vi "trim_string_of_wspaces_and_quotes.vi"(4 "String in":string, 5 "Remove quotes (Remove All)":u16(ring) items=["Remove All Quotes", "Remove Single Quotes", "Remove Double Quotes", "Remove None"]) -> (1 "String out":string)   [LabVIEW 2014, in "rszvl_rsidr_core.lvlib"]
uses:
  rszvl_rsidr_core.lvlib
  Match Regular Expression.xnode
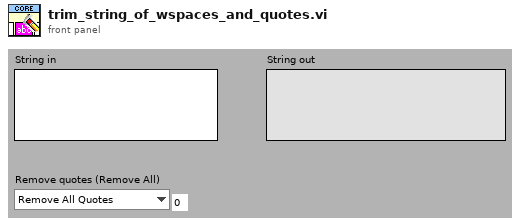
[diagram p1: front panel]
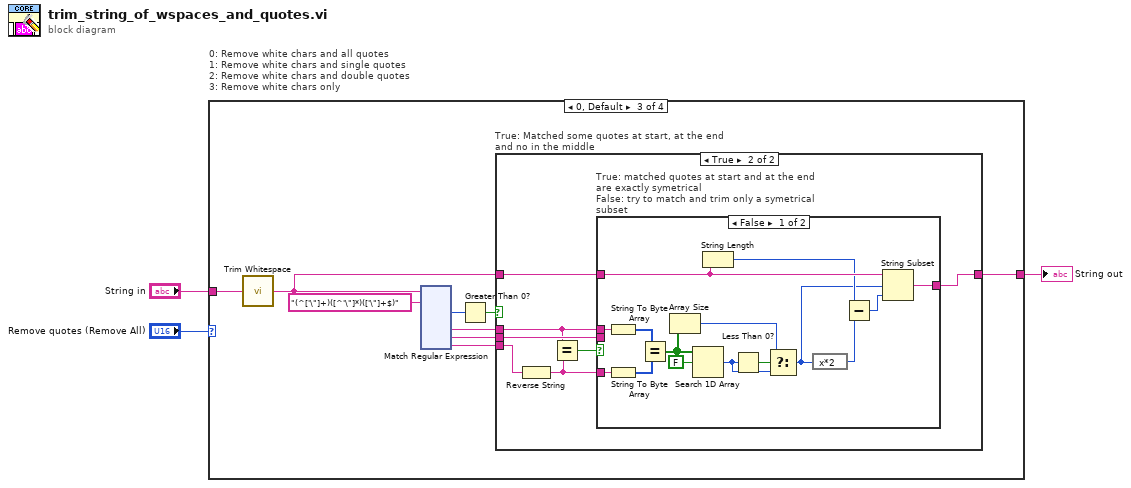
[diagram p0: block diagram]
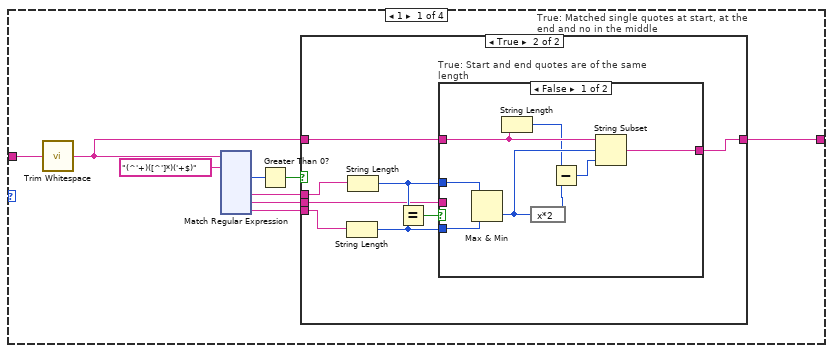
[diagram p2: hidden frame]
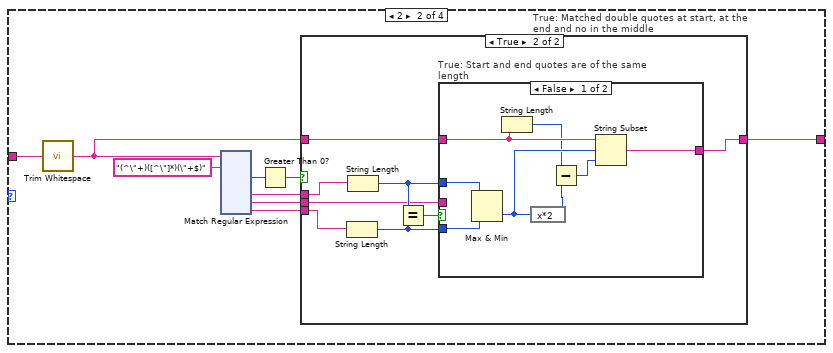
[diagram p5: hidden frame]
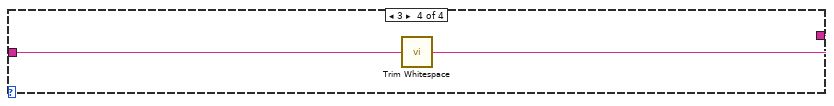
[diagram p10: hidden frame]
diagram:
  n1 = case "0: Remove white chars and all quotes\n1: Remove white chars and single quotes\n2: Remove white chars and double quotes\n3: Remove white chars only" shown="0, Default" "Remove quotes (Remove All)" {
    tunnel: "String in" -> [w12 w154 w296 w437]
    tunnel: [w5 w148 w288 w436] -> w1
    frame 1 {
      n2 = call "Trim Whitespace.vi"("string"=w12) -> ("trimmed string"=w4:string)  [unwired: 1 in]
      n3 = xnode ("Match Regular Expression")("input string"=w4, "regular expression"="(^'+)([^']*)('+$)") -> ("offset past match"=w10:i32, "submatch 1"=w8:string, "submatch 2"=w7:string, "submatch 3"=w6:string)  [unwired: 4 in, 4 out]
      n4 = Greater Than 0?(x=w10) -> (x > 0?=w9:bool)
      n5 = case "True: Matched single quotes at start, at the end and no in the middle" shown="True" w9 {
        tunnel: w8 -> [_ w20]
        tunnel: w7 -> [_ w16]
        tunnel: w6 -> [_ w21]
        tunnel: [w13 w15] -> w5
        tunnel: w4 -> [w13 w14]
        frame False {
        }
        frame True {
          n6 = String Length(string=w21) -> (length=w17:i32)
          n7 = String Length(string=w20) -> (length=w18:i32)
          n8 = Equal?(x=w18, y=w17) -> (x = y?=w19:bool)
          n9 = case "True: Start and end quotes are of the same length" shown="False" w19 {
            tunnel: w18 -> [w29 _]
            tunnel: w17 -> [w28 _]
            tunnel: w16 -> [_ w30]
            tunnel: [w22 w30] -> w15
            tunnel: w14 -> [w27 _]
            frame False {
              n10 = Max & Min(x=w29, y=w28) -> (min(x,y)=w26:i32)  [unwired: 1 out]
              n11 = String Length(string=w27) -> (length=w25:i32)
              n12 = expression code="x*2"(w26) -> (w24:i32)
              n13 = Subtract(x=w25, y=w24) -> (x-y=w23:i32)
              n14 = String Subset(string=w27, offset (0)=w26, length (rest)=w23) -> (substring=w22:string)
            }
            frame True {
            }
          }
        }
      }
    }
    frame 2 {
      n15 = call "Trim Whitespace.vi"("string"=w154) -> ("trimmed string"=w147:string)  [unwired: 1 in]
      n16 = xnode ("Match Regular Expression")("input string"=w147, "regular expression"="(^\"+)([^\"]*)(\"+$)") -> ("offset past match"=w153:i32, "submatch 1"=w151:string, "submatch 2"=w150:string, "submatch 3"=w149:string)  [unwired: 4 in, 4 out]
      n17 = Greater Than 0?(x=w153) -> (x > 0?=w152:bool)
      n18 = case "True: Matched double quotes at start, at the end and no in the middle" shown="True" w152 {
        tunnel: w151 -> [_ w162]
        tunnel: w150 -> [_ w158]
        tunnel: w149 -> [_ w163]
        tunnel: [w155 w157] -> w148
        tunnel: w147 -> [w155 w156]
        frame False {
        }
        frame True {
          n19 = String Length(string=w163) -> (length=w159:i32)
          n20 = String Length(string=w162) -> (length=w160:i32)
          n21 = Equal?(x=w160, y=w159) -> (x = y?=w161:bool)
          n22 = case "True: Start and end quotes are of the same length" shown="False" w161 {
            tunnel: w160 -> [w171 _]
            tunnel: w159 -> [w170 _]
            tunnel: w158 -> [_ w172]
            tunnel: [w164 w172] -> w157
            tunnel: w156 -> [w169 _]
            frame False {
              n23 = Max & Min(x=w171, y=w170) -> (min(x,y)=w168:i32)  [unwired: 1 out]
              n24 = String Length(string=w169) -> (length=w167:i32)
              n25 = expression code="x*2"(w168) -> (w166:i32)
              n26 = Subtract(x=w167, y=w166) -> (x-y=w165:i32)
              n27 = String Subset(string=w169, offset (0)=w168, length (rest)=w165) -> (substring=w164:string)
            }
            frame True {
            }
          }
        }
      }
    }
    frame 0, Default {
      n28 = call "Trim Whitespace.vi"("string"=w296) -> ("trimmed string"=w289:string)  [unwired: 1 in]
      n29 = xnode ("Match Regular Expression")("input string"=w289, "regular expression"="(^['\"]+)([^'\"]*)(['\"]+$)") -> ("offset past match"=w294:i32, "submatch 1"=w292:string, "submatch 2"=w291:string, "submatch 3"=w290:string)  [unwired: 4 in, 4 out]
      n30 = Greater Than 0?(x=w294) -> (x > 0?=w293:bool)
      n31 = case "True: Matched some quotes at start, at the end and no in the middle" shown="True" w293 {
        tunnel: w292 -> [_ w298]
        tunnel: w291 -> [_ w303]
        tunnel: w290 -> [_ w300]
        tunnel: [w297 w302] -> w288
        tunnel: w289 -> [w297 w301]
        frame False {
        }
        frame True {
          n32 = Reverse String(1:w300) -> (0:w299:string)
          n33 = Equal?(x=w298, y=w299) -> (x = y?=w304:bool)
          n34 = case "True: matched quotes at start and at the end are exactly symetrical\nFalse: try to match and trim only a symetrical subset" shown="False" w304 {
            tunnel: w303 -> [_ w320]
            tunnel: [w316 w320] -> w302
            tunnel: w301 -> [w319 _]
            tunnel: w299 -> [w314 _]
            tunnel: w298 -> [w315 _]
            frame False {
              n35 = String To Byte Array(string=w315) -> (unsigned byte array=w313:u8[])
              n36 = String To Byte Array(string=w314) -> (unsigned byte array=w312:u8[])
              n37 = Equal?(x=w313, y=w312) -> (x = y?=w307:bool[])
              n38 = Array Size(array=w307) -> (size(s)=w306:i32)
              n39 = Search 1D Array(1D array=w307, element=FALSE) -> (index of element=w309:i32)  [unwired: 1 in]
              n40 = String Length(string=w319) -> (length=w318:i32)
              n41 = Less Than 0?(x=w309) -> (x < 0?=w310:bool)
              n42 = Select(t=w306, s=w310, f=w309) -> (s? t:f=w308:i32)
              n43 = expression code="x*2"(w308) -> (w305:i32)
              n44 = Subtract(x=w318, y=w305) -> (x-y=w317:i32)
              n45 = String Subset(string=w319, offset (0)=w308, length (rest)=w317) -> (substring=w316:string)
            }
            frame True {
            }
          }
        }
      }
    }
    frame 3 {
      n46 = call "Trim Whitespace.vi"("string"=w437) -> ("trimmed string"=w436:string)  [unwired: 1 in]
    }
  }
  "String out" <- w1
